vi "slope.vi"(11 "input":cluster{dbl[], dbl[]}) -> (3 "output":cluster{dbl[], dbl[]})   [LabVIEW 2014]
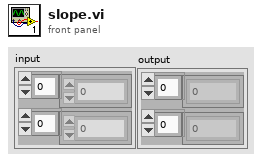
[diagram p1: front panel]
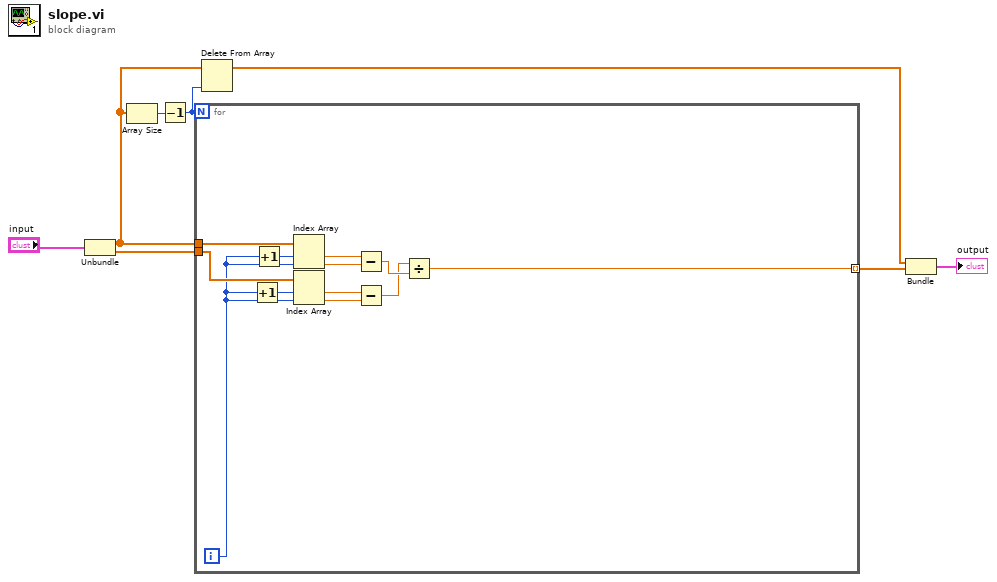
[diagram p0: block diagram]
diagram:
  n1 = Unbundle("input") -> (w4:dbl[], w6:dbl[])
  n2 = Array Size(array=w4) -> (size(s)=w7:i32)
  n3 = Decrement(x=w7) -> (x-1=w1:i32)
  n4 = for {
    N: w1 -> [_]
    tunnel: w4 -> [w20]
    tunnel: w6 -> [w19]
    tunnel: [w9] -> w5 mode=indexing
    i -> [w18]
    n5 = Increment(x=w18) -> (x+1=w16:i32)
    n6 = Increment(x=w18) -> (x+1=w17:i32)
    n7 = Index Array(array=w20, index #1=w17, index #2=w18) -> (element #1=w15:dbl, element #2=w14:dbl)
    n8 = Index Array(array=w19, index #1=w16, index #2=w18) -> (element #1=w13:dbl, element #2=w12:dbl)
    n9 = Subtract(x=w15, y=w14) -> (x-y=w11:dbl)
    n10 = Subtract(x=w13, y=w12) -> (x-y=w10:dbl)
    n11 = Divide(x=w10, y=w11) -> (x/y=w9:dbl)
  }
  n12 = Delete From Array(array=w4, index=w1) -> (array with subset deleted=w2:dbl[])  [unwired: 1 in, 1 out]
  n13 = Bundle(w2, w5) -> (→"output":cluster{dbl[], dbl[]})  [unwired: 1 in]
